vi "Drive_Loop_Control_Loop.vi"(10 "Init Period":i64, 11 "Drive DevRef In":T2={"Sensor Data"={"Gyro Data"={"Gyro RT FIFO"=refnum, "Gyro Current"=0.0, "Gyro Hold"=0.0}, "Encoder Data"={"Encoder RT FIFO"=refnum, "Encoder Current"=0.0, "Encoder Hold"=0.0}, "Camera Data"={"Camera RT FIFO"=refnum, "Camera Current"={" Angle"=0.0, "Valid"=FALSE}}}, "PID Update"=refnum, "RobotDriveDevRef"={"DevStatus"={"status"=FALSE, "code"=0, "source"=""}, "Motors[]"=[], "Square Inputs"=FALSE, "Max Output"=1.0}, "Drive Train"=enum."Tank Drive 2 Motor", "Valid Commands"=[], "Drive Comand Notifier"=refnum, "Command Finished?"=refnum, "Command Canceled"=refnum}) -> ()   [LabVIEW 2016]
doc: "Help file written by FRC Team 836 - The RoboBees\n\nThis VI combines movment commands with various sensor inputs to control the robot as desired.\n\nThis VI uses VIs & Controls from Worcestor Polytechnic Institure (WPI) located in folder:\nC:\\Program Files (x86)\\National Instruments\\LabVIEW 2015\\vi.lib\\Rock Robotics\\WPI\\RobotDrive\n\nThe RobotDrive VI from WPI does the actual moving of the robot. The RobotDriveDevRef control\nwill pass commands to the WPI VI \"WPI_RobotDriveMotors\" via the WPI VI \"WPI_RobotDriveTankDrive\" to acutate the motors.\n\nThe RT FIFOs must be initialized using the \"Drive_Loop_Initialize_w_Help\" VI."
uses:
  <userlib>/836-libraries/Drive/Drive_Code_V2/Drive_Code_Support/Drive_Code_Bundle.ctl
  <userlib>/836-libraries/Drive/Drive_Code_V2/Drive_Code_Support/SensorTypedefs/Sensor_Cluster.ctl
  <userlib>/836-libraries/Drive/Drive_Code_V2/Drive_Code_Support/SensorTypedefs/Camera_Cluster.ctl
  <userlib>/836-libraries/Drive/Drive_Code_V2/Drive_Code_Support/PidClusters/Drive_Code_PID_Bundle.ctl
  <vilib>/Rock Robotics/WPI/RobotDrive/WPI_RobotDriveDevRef.ctl
  <vilib>/Rock Robotics/WPI/MotorControl/WPI_MotorControlDeviceRef.ctl
  <vilib>/Rock Robotics/WPI/MotorControl/WPI_MotorControlType.ctl
  <vilib>/Rock Robotics/SystemInterfaces/DIO/FPGA_DIOPWMChannel.ctl
  <vilib>/Rock Robotics/WPI/PWM/WPI_PWMDeadband.ctl
  <userlib>/836-libraries/Drive/Drive_Code_V2/Drive_Code_Support/DriveTrains/Drive_Trains.ctl
  <userlib>/836-libraries/Drive/Drive_Code_V2/Drive_Code_Support/Command_Sends/Drive_Code_Command_Type.ctl
  <userlib>/836-libraries/Drive/Drive_Code_V2/Drive_Code_Support/Command_Sends/Drive_Code_Command_List.ctl
  <vilib>/Platform/TimedLoop/XDataNode/timing_clust.ctl
  <vilib>/Platform/TimedLoop/XDataNode/nitl_modes.ctl
  <vilib>/Platform/TimedLoop/XDataNode/wakeup.ctl
  <userlib>/836-libraries/Drive/Drive_Code_V2/Drive_Code_Support/DriveTrains/Drive_Values.ctl
  <userlib>/836-libraries/Drive/Drive_Code_V2/Drive_Code_Support/Command_Sends/CommandTypeInfo/DriveContinuousParam.ctl
  <userlib>/836-libraries/Drive/Drive_Code_V2/Drive_Code_Support/Command_Sends/CommandTypeInfo/AngleInfo.ctl
  <userlib>/836-libraries/Drive/Drive_Code_V2/Drive_Code_Support/Command_Sends/CommandTypeInfo/TurnParam.ctl
  <userlib>/836-libraries/Drive/Drive_Code_V2/Drive_Code_Support/Command_Sends/CommandTypeInfo/DriveDistanceParam.ctl
  <userlib>/836-libraries/Drive/Drive_Code_V2/Drive_Code_Support/Command_Sends/CommandTypeInfo/DistanceInfo.ctl
  <userlib>/836-libraries/Drive/Drive_Code_V2/Drive_Code_Support/Command_Sends/CommandTypeInfo/ApproachCameraParam.ctl
  <userlib>/836-libraries/Drive/Drive_Code_V2/Drive_Code_Support/Command_Sends/CommandTypeInfo/UpdatePeriodParam.ctl
  <vilib>/addons/control/pid/pid.llb/PID (DBL).vi
  <vilib>/platform/TimedLoop/XDataNode/XDataNode.xnode
  <vilib>/Platform/TimedLoop/XDataNode/XDNodeRunTimeDep.lvlib
  <vilib>/addons/control/pid/NI_PID_pid.lvlib
panel:
  in  "Init PID Gains":T1={"Yaw, Driving Straight"={"proportional gain (Kc)"=1.0, "integral time (Ti, min)"=0.01, "derivative time (Td, min)"=0.0}, "Yaw, Holding Still"={"proportional gain (Kc)"=1.0, "integral time (Ti, min)"=0.01, "derivative time (Td, min)"=0.0}, "Distance, Driving Straight"={"proportional gain (Kc)"=1.0, "integral time (Ti, min)"=0.01, "derivative time (Td, min)"=0.0}, "Distance, Holding Still"={"proportional gain (Kc)"=1.0, "integral time (Ti, min)"=0.01, "derivative time (Td, min)"=0.0}}
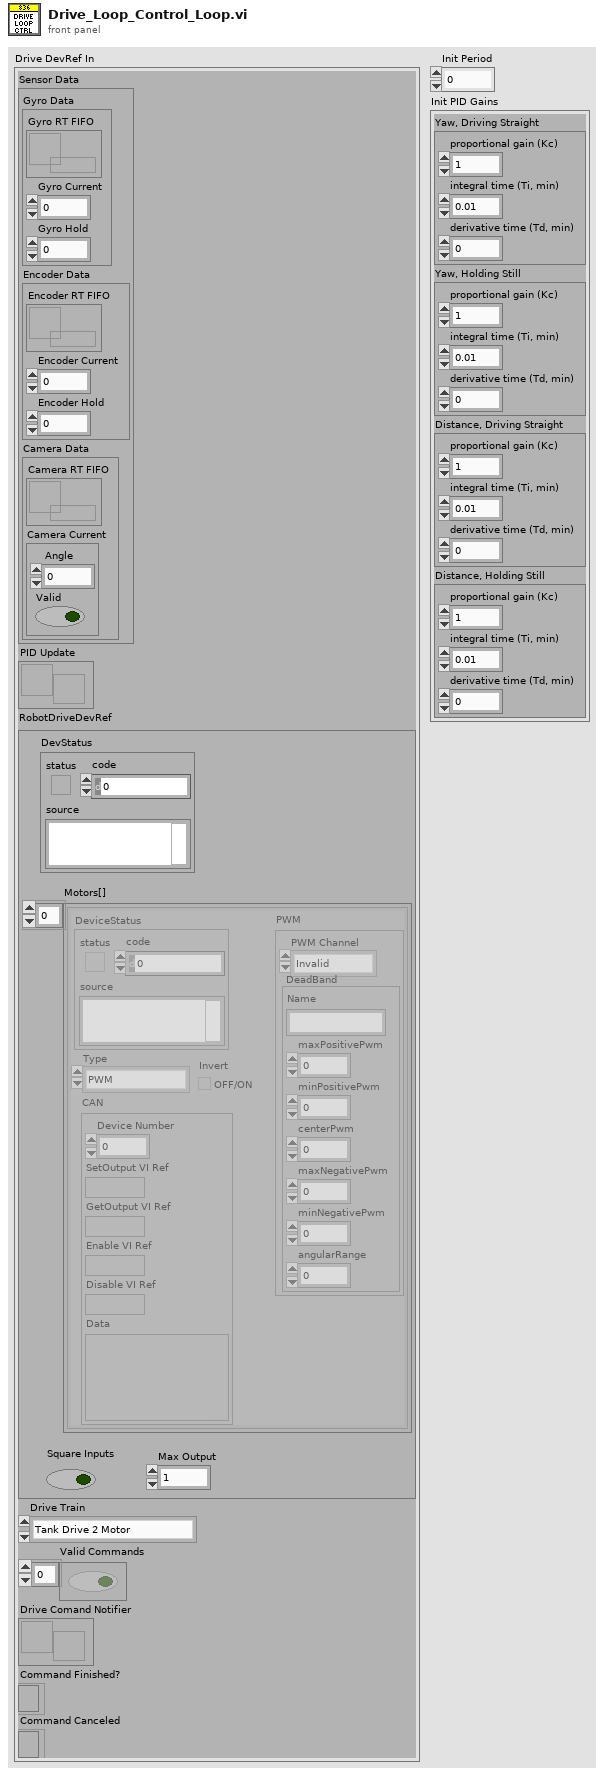
[diagram p1: front panel]
types:
  T1 = typedef "Drive_Code_PID_Bundle.ctl" = cluster{"Yaw, Driving Straight":cluster{"proportional gain (Kc)":dbl, "integral time (Ti, min)":dbl, "derivative time (Td, min)":dbl}, "Yaw, Holding Still":cluster{"proportional gain (Kc)":dbl, "integral time (Ti, min)":dbl, "derivative time (Td, min)":dbl}, "Distance, Driving Straight":cluster{"proportional gain (Kc)":dbl, "integral time (Ti, min)":dbl, "derivative time (Td, min)":dbl}, "Distance, Holding Still":cluster{"proportional gain (Kc)":dbl, "integral time (Ti, min)":dbl, "derivative time (Td, min)":dbl}}
  T2 = typedef "Drive_Code_Bundle.ctl" = cluster{"Sensor Data":T3, "PID Update":refnum<notifier>, "RobotDriveDevRef":T5, "Drive Train":T10, "Valid Commands":bool[], "Drive Comand Notifier":refnum<notifier>, "Command Finished?":refnum<k4>, "Command Canceled":refnum<k4>}
  T3 = typedef "Sensor_Cluster.ctl" = cluster{"Gyro Data":cluster{"Gyro RT FIFO":refnum<k33>, "Gyro Current":dbl, "Gyro Hold":dbl}, "Encoder Data":cluster{"Encoder RT FIFO":refnum<k33>, "Encoder Current":dbl, "Encoder Hold":dbl}, "Camera Data":cluster{"Camera RT FIFO":refnum<k33>, "Camera Current":T4}}
  T4 = typedef "Camera_Cluster.ctl" = cluster{" Angle":dbl, "Valid":bool}
  T5 = typedef "WPI_RobotDriveDevRef.ctl" = cluster{"DevStatus":errorcluster, "Motors[]":T6[], "Square Inputs":bool, "Max Output":dbl}
  T6 = typedef "WPI_MotorControlDeviceRef.ctl" = cluster{"DeviceStatus":errorcluster, "Type":T7, "PWM":cluster{"PWM Channel":T8, "DeadBand":T9}, "CAN":cluster{"Device Number":u8, "SetOutput VI Ref":variant, "GetOutput VI Ref":variant, "Enable VI Ref":variant, "Disable VI Ref":variant, "Data":variant}, "Invert":bool}
  T7 = typedef "WPI_MotorControlType.ctl" = enum16{"PWM", "CAN"}
  T8 = typedef "FPGA_DIOPWMChannel.ctl" = enum8{"PWM 0", "PWM 1", "PWM 2", "PWM 3", "PWM 4", "PWM 5", "PWM 6", "PWM 7", "PWM 8", "PWM 9", "PWM MXP 0", "PWM MXP 1", "PWM MXP 2", "PWM MXP 3", "PWM MXP 4", "PWM MXP 5", "PWM MXP 6", "PWM MXP 7", "PWM MXP 8", "PWM MXP 9", "Invalid"}
  T9 = typedef "WPI_PWMDeadband.ctl" = cluster{"Name":string, "maxPositivePwm":i32, "minPositivePwm":i32, "centerPwm":i32, "maxNegativePwm":i32, "minNegativePwm":i32, "angularRange":u16}
  T10 = typedef "Drive_Trains.ctl" = enum16{"Tank Drive 2 Motor", "Tank Drive 4 Motor", "Mecanum Drive", "Kiwi Drive"}
  T11 = typedef "Drive_Code_Command_List.ctl" = enum16{"Do Nothing", "Tank Drive", "Drive Continuous", "Turn", "Drive Distance", "Hold Position", "Hold Yaw", "Follow Camera", "Turn to Camera", "Approach Camera", "PID Update", "Cheesy Drive", "Update Period"}
  T12 = typedef "Drive_Code_Command_Type.ctl" = cluster{"Command":T11, "Command Params":variant}
  T13 = typedef "XDNodeRunTimeDep.lvlib/timing_clust.ctl" = cluster{"Expected End [f-1]":u64, "Actual End [f-1]":u64, "Finished Late? [f-1]":bool, "Expected End [i-1]":u64, "Actual End [i-1]":u64, "Finished Late? [i-1]":bool, "Expected Start [i]":u64, "Actual Start [i]":u64, "Expected Start [f]":u64, "Actual Start [f]":u64, "Source Name":string, "Structure Name":string, "Period":i64, "Deadline":i64, "Offset":i64, "Start":i64, "Priority":i32, "Timeout":i32, "Mode":T14, "Wakeup Reason":T15, "Error":errorcluster, "Source Type":string, "Secondary Source Type":string, "Global End Time":u64, "Global Start Time":u64, "Frame Duration":u64, "Iteration Duration":u64, "Assigned CPU":i32, "I/O Scan Engine Mode":u32}
  T14 = typedef "XDNodeRunTimeDep.lvlib/nitl_modes.ctl" = enum32{"No Change", "Process missed periods, maintain original phase", "Discard missed periods, maintain original phase", "Process missed periods, ignore original phase", "Discard missed periods, ignore original phase"}
  T15 = typedef "XDNodeRunTimeDep.lvlib/wakeup.ctl" = enum32{"Normal", "Aborted", "Asynchronous wakeup", "Timing source error", "Timed loop error", "Timeout"}
  T16 = typedef "Drive_Values.ctl" = cluster{"Right":dbl, "Left":dbl, "Throttle":dbl, "Wheel":dbl, "Rotation":dbl, "X":dbl, "Y":dbl}
  T17 = typedef "DriveContinuousParam.ctl" = cluster{"Max Turn Power":dbl, "Angle To Drive At":T18, "Foward Power":dbl}
  T18 = typedef "AngleInfo.ctl" = cluster{"Angle":dbl, "Angle Absolute?":bool}
  T19 = typedef "TurnParam.ctl" = cluster{"Max Power":dbl, "Angle To Turn To":T18}
  T20 = typedef "DriveDistanceParam.ctl" = cluster{"Max Turn Power":dbl, "Distance To Drive":T21, "Angle To Drive At":T18, "Max Forward Power":dbl}
  T21 = typedef "DistanceInfo.ctl" = cluster{"Distance":dbl, "Distance Absolute?":bool}
  T22 = typedef "ApproachCameraParam.ctl" = cluster{"Max Turn Power":dbl, "Distance To Drive":T21, "Max Forward Power":dbl}
  T23 = typedef "UpdatePeriodParam.ctl" = cluster{"Period":i64}
  T24 = cluster{"Gyro RT FIFO":refnum<k33>, "Gyro Current":dbl, "Gyro Hold":dbl}
  T25 = cluster{"Encoder RT FIFO":refnum<k33>, "Encoder Current":dbl, "Encoder Hold":dbl}
  T26 = cluster{"Camera RT FIFO":refnum<k33>, "Camera Current":T4}
  T27 = typedef "DrivePidInputs.ctl" = cluster{"EncoderPID":T28, "YawPID":T28}
  T28 = typedef "PidInputs.ctl" = cluster{"Setpoint":dbl, "Process":dbl}
  T29 = typedef "DrivePidRange.ctl" = cluster{"Encoder PID Range":T30, "Yaw PID Range":T30}
  T30 = typedef "PidRange.ctl" = cluster{"Max":dbl, "Min":dbl}
  T31 = cluster{"proportional gain (Kc)":dbl, "integral time (Ti, min)":dbl, "derivative time (Td, min)":dbl}
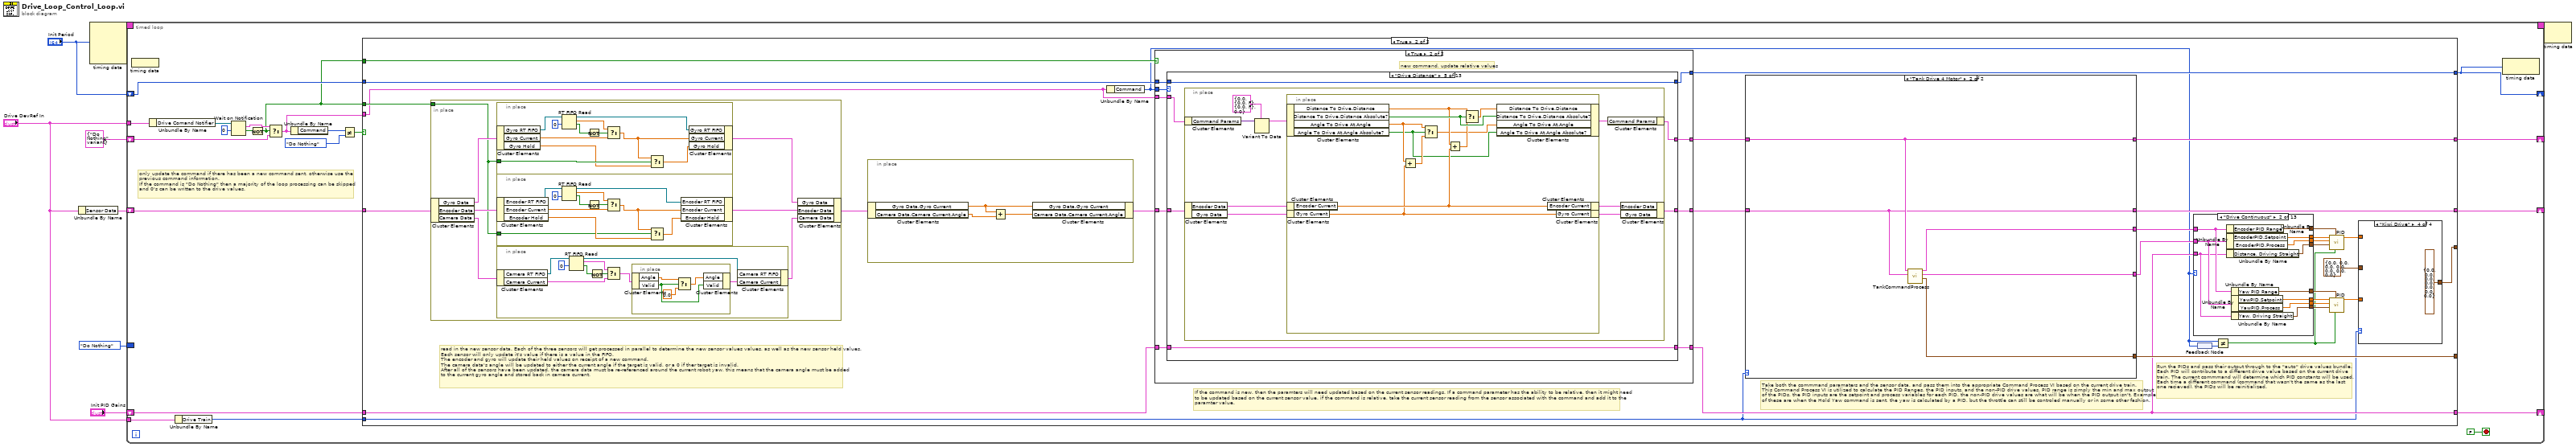
[diagram p0: block diagram]
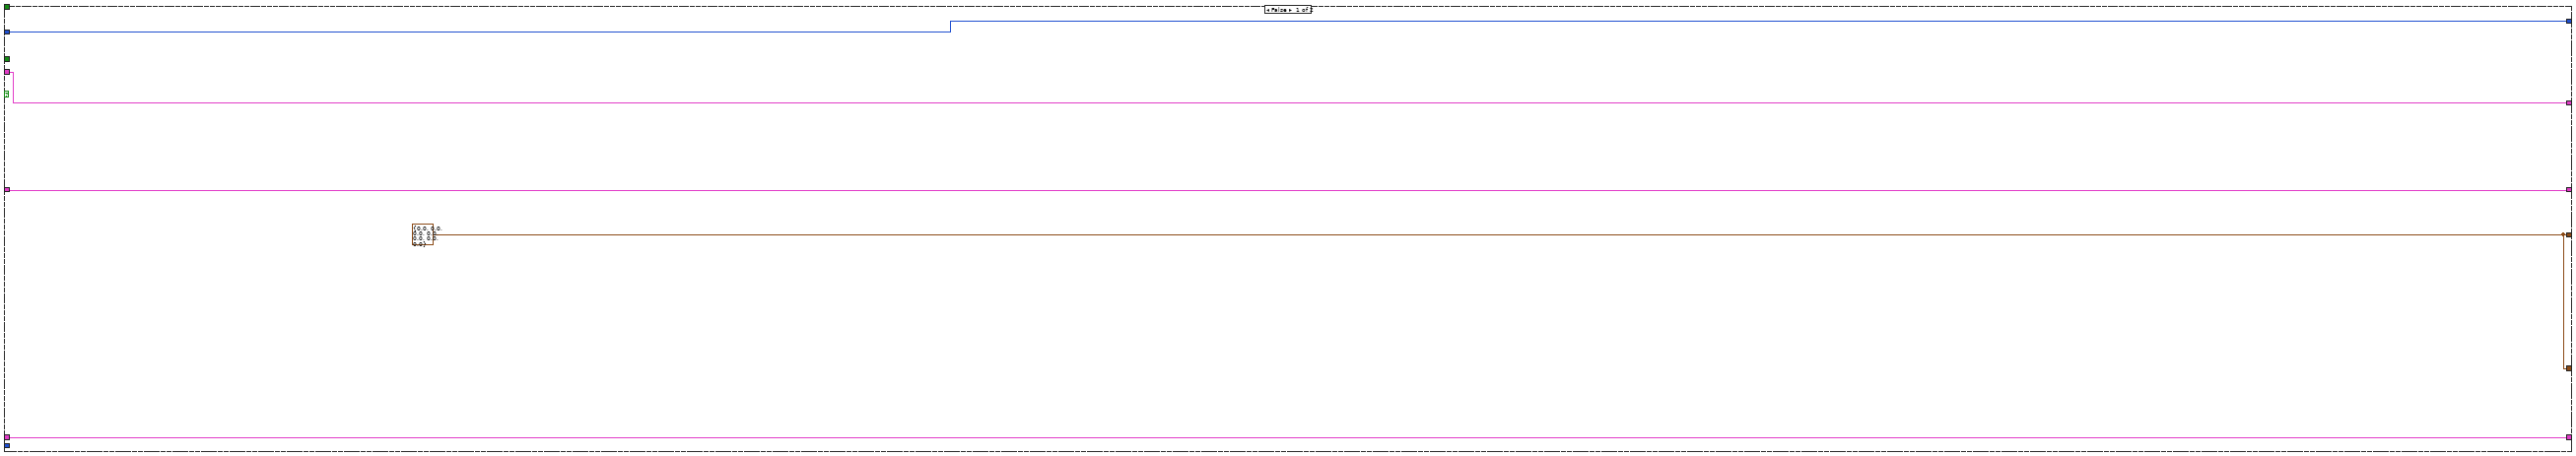
[diagram p2: hidden frame]
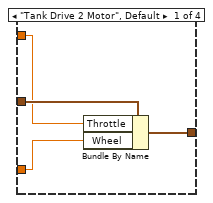
[diagram p3: hidden frame]
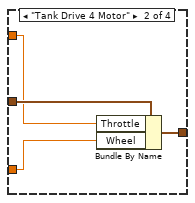
[diagram p4: hidden frame]
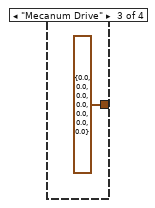
[diagram p5: hidden frame]
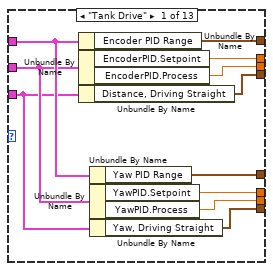
[diagram p6: hidden frame]
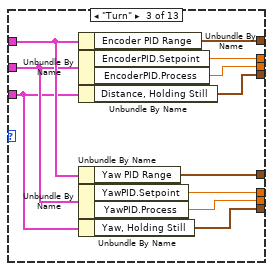
[diagram p7: hidden frame]
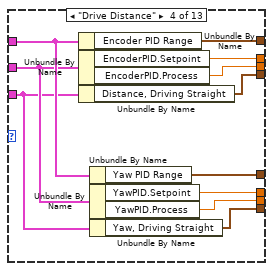
[diagram p8: hidden frame]
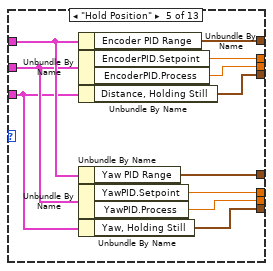
[diagram p9: hidden frame]
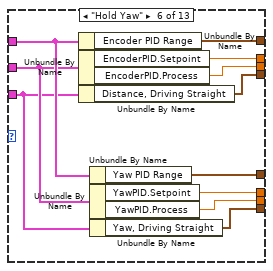
[diagram p10: hidden frame]
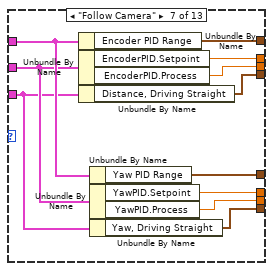
[diagram p11: hidden frame]
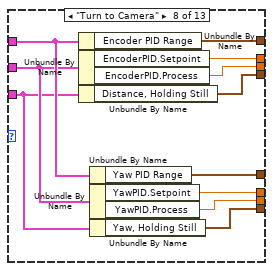
[diagram p12: hidden frame]
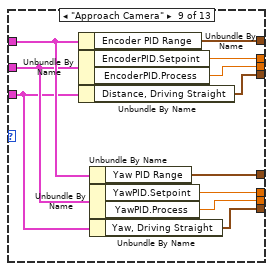
[diagram p13: hidden frame]
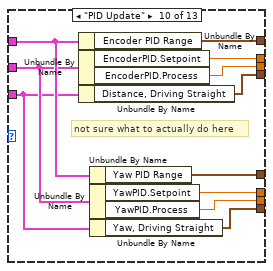
[diagram p14: hidden frame]
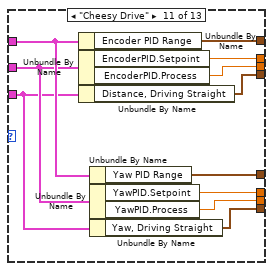
[diagram p15: hidden frame]
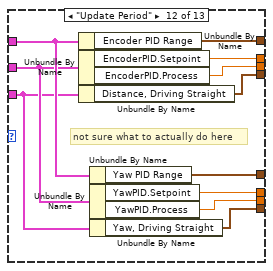
[diagram p16: hidden frame]
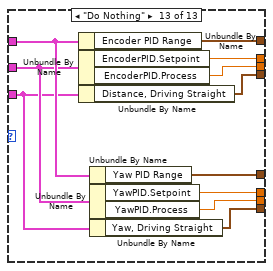
[diagram p17: hidden frame]
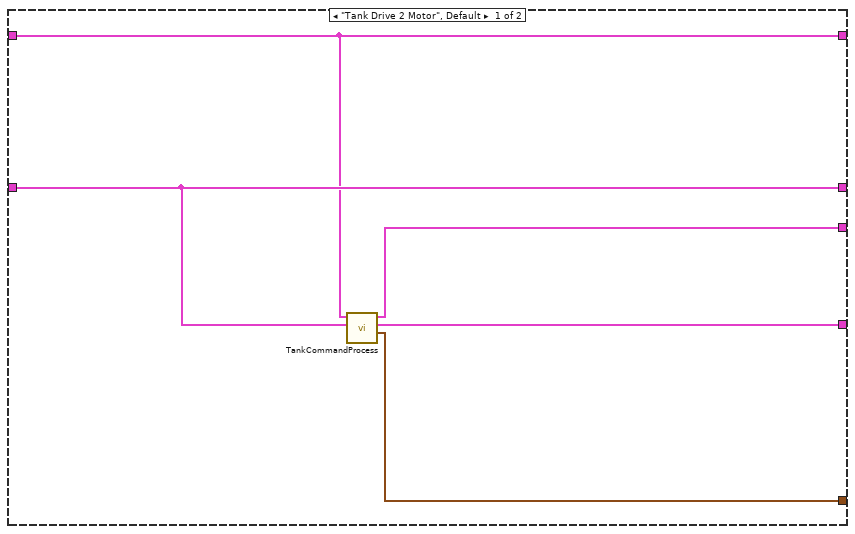
[diagram p18: hidden frame]
diagram:
  n1 = Unbundle By Name("Drive DevRef In") -> ("Sensor Data"=w3:T3)
  n2 = node-c288("Init Period") -> (w8:T13)  [unwired: 3 in]
  n3 = timed-loop {
    timing: w8 -> [_]
    timing-out: [_] -> w7
    shift-right: [w17] -> _
    shift-left: "Init Period" -> [w18]
    tunnel: "Drive DevRef In" -> [w20]
    shift-right: [w16] -> _
    shift-left: T12 {"Command"=enum."Do Nothing", "Command Params"=variant} ("Command Type") -> [w24]
    shift-right: [w13] -> _
    shift-left: "Init PID Gains" -> [w14]
    shift-right: [w15] -> _
    shift-left: w3 -> [w19]
    tunnel: "Drive DevRef In" -> [w10]
    border: Drive_Code_Command_List."Do Nothing" ("Command") -> [_]
    stop <- FALSE stop-if-true
    # "only update the command if there has been a new command sent, otherwise use the\nprevious command information.\nIf the command is \"Do Nothing\" then a majority of the loop processing can be skipped\nand 0's can be written to the drive values."
    n4 = node-c288() -> ()  [unwired: 1 in]
    n5 = Unbundle By Name(w20) -> ("Drive Comand Notifier"=w28:refnum<notifier>)
    n6 = Unbundle By Name(w10) -> ("Drive Train"=w9:T10)
    n7 = Wait on Notification(notifier=w28, timeout in ms (-1)=0) -> (notification=w25:T12, timed out?=w26:bool)  [unwired: 2 in, 2 out]
    n8 = Not(x=w26) -> (.not. x?=w11:bool)
    n9 = Select(t=w25, s=w11, f=w24) -> (s? t:f=w21:T12)
    n10 = Unbundle By Name(w21) -> ("Command"=w12:T11)
    n11 = Not Equal?(x=w12, y=Drive_Code_Command_List."Do Nothing") -> (x != y?=w22:bool)
    n12 = case shown="True" w22 {
      tunnel: [w30 w35] -> _
      tunnel: w21 -> [w33 w64]
      tunnel: w11 -> [_ w67]
      tunnel: w19 -> [w32 w66]
      tunnel: w18 -> [w34 w65]
      tunnel: [w34 w63] -> w17
      tunnel: [w33 w57] -> w16
      tunnel: [w32 w56] -> w15
      tunnel: w14 -> [w31 w62]
      tunnel: [w31 w48] -> w13
      tunnel: w11 -> [_ w43]
      tunnel: w9 -> [_ w38]
      tunnel: [w30 w55] -> _
      frame False {
        w30 = T16 {"Right"=0.0, "Left"=0.0, "Throttle"=0.0, "Wheel"=0.0, "Rotation"=0.0, "X"=0.0, "Y"=0.0}
      }
      frame True {
        # "Run the PIDs and pass their output through to the \"auto\" drive values bundle.\nEach PID will contribute to a different drive value based on the current drive\ntrain. The current commmand will determine which PID constants will be used.\nEach time a different command (command that wasn't the same as the last \none recieved), the PIDs will be reinitialized."
        # "Take both the commmand paramaters and the sensor data, and pass them into the appropriate Command Process VI based on the current drive train.\nThis Command Process VI is utilized to calculate the PID Ranges, the PID inputs, and the non-PID drive values. PID range is simply the min and max output\nof the PIDs, the PID inputs are the setpoint and process variables for each PID, the non-PID drive values are what will be when the PID output isn't. Examples\nof these are when the Hold Yaw command is sent, the yaw is calculated by a PID, but the throttle can still be controled manually or in some other fashion."
        # "If the command is new, then the paramters will need updated based on the current sensor readings. If a command parameter has the ability to be relative, then it might need\nto be updated based on the current sensor value. if the command is relative, take the current sensor reading from the sensor associated with the command and add it to the\nparamter value."
        # "read in the new sensor data. Each of the three sensors will get processed in parallel to determine the new sensor values values, as well as the new sensor held values.\nEach sensor will only update it's value if there is a value in the FIFO.\nThe encoder and gyro will update their held values on receipt of a new command.\nThe camera data's angle will be updated to either the current angle if the target is valid, or a 0 if ther target is invalid.\nAfter all of the sensors have been updated, the camera data must be re-referenced around the current robot yaw, this means that the camera angle must be added\nto the current gyro angle and stored back in camera current."
        n13 = in-place {
          in-place-border: w67 -> [w366]
          n14 = in-place-cluster #1(w66) -> ("Gyro Data"=w372:T24, "Encoder Data"=w370:T25, "Camera Data"=w368:T26)
          n15 = in-place {
            in-place-border: w366 -> [w399]
            n16 = in-place-cluster #2(w372) -> ("Gyro RT FIFO"=w407:refnum<k33>, "Gyro Current"=w401:dbl, "Gyro Hold"=w397:dbl)
            n17 = RT FIFO Read(0:w407, 2:0 ("timeout in ms (0)")) -> (8:w405:refnum<k33>, 9:w403:dbl, 10:w404:bool)  [unwired: 2 in, 2 out]
            n18 = Not(x=w404) -> (.not. x?=w402:bool)
            n19 = Select(t=w403, s=w402, f=w401) -> (s? t:f=w398:dbl)
            n20 = Select(t=w398, s=w399, f=w397) -> (s? t:f=w400:dbl)
            n21 = in-place-cluster #2("Gyro RT FIFO"=w405, "Gyro Current"=w398, "Gyro Hold"=w400) -> (w371:T24)
          }
          n22 = in-place {
            in-place-border: w366 -> [w386]
            n23 = in-place-cluster #3(w370) -> ("Encoder RT FIFO"=w396:refnum<k33>, "Encoder Current"=w390:dbl, "Encoder Hold"=w387:dbl)
            n24 = RT FIFO Read(0:w396, 2:0 ("timeout in ms (0)")) -> (8:w394:refnum<k33>, 9:w392:dbl, 10:w393:bool)  [unwired: 2 in, 2 out]
            n25 = Not(x=w393) -> (.not. x?=w391:bool)
            n26 = Select(t=w392, s=w391, f=w390) -> (s? t:f=w388:dbl)
            n27 = Select(t=w388, s=w386, f=w387) -> (s? t:f=w389:dbl)
            n28 = in-place-cluster #3("Encoder RT FIFO"=w394, "Encoder Current"=w388, "Encoder Hold"=w389) -> (w369:T25)
          }
          n29 = in-place {
            n30 = in-place-cluster #4(w368) -> ("Camera RT FIFO"=w381:refnum<k33>, "Camera Current"=w375:T4)
            n31 = RT FIFO Read(0:w381, 2:0 ("timeout in ms (0)")) -> (8:w379:refnum<k33>, 9:w376:T4, 10:w378:bool)  [unwired: 2 in, 2 out]
            n32 = Not(x=w378) -> (.not. x?=w377:bool)
            n33 = Select(t=w376, s=w377, f=w375) -> (s? t:f=w374:T4)
            n34 = in-place {
              n35 = in-place-cluster #5(w374) -> ("Angle"=w385:dbl, "Valid"=w383:bool)
              n36 = Select(t=w385, s=w383, f=0.0) -> (s? t:f=w384:dbl)
              n37 = in-place-cluster #5("Angle"=w384, "Valid"=w383) -> (w373:T4)
            }
            n38 = in-place-cluster #4("Camera RT FIFO"=w379, "Camera Current"=w373) -> (w367:T26)
          }
          n39 = in-place-cluster #1("Gyro Data"=w371, "Encoder Data"=w369, "Camera Data"=w367) -> (w59:T3)
        }
        n40 = in-place {
          n41 = in-place-cluster #6(w59) -> ("Gyro Data.Gyro Current"=w223:dbl, "Camera Data.Camera Current.Angle"=w221:dbl)
          n42 = Add(x=w223, y=w221) -> (x+y=w222:dbl)
          n43 = in-place-cluster #6("Gyro Data.Gyro Current"=w223, "Camera Data.Camera Current.Angle"=w222) -> (w58:T3)
        }
        n44 = Unbundle By Name(w64) -> ("Command"=w41:T11)
        n45 = case shown="True" w43 {
          tunnel: w65 -> [w234 w246]
          tunnel: w58 -> [w236 w245]
          tunnel: w41 -> [_ w244]
          tunnel: w64 -> [w237 w243]
          tunnel: [w234 w242] -> w63
          tunnel: [w236 w241] -> w60
          tunnel: [w237 w240] -> w61
          tunnel: [w235 w239] -> w48
          tunnel: w62 -> [w235 w238]
          frame False {
          }
          frame True {
            # "new command, update relative values"
            n46 = case shown="\"Drive Distance\"" w244 {
              tunnel: w246 -> [w250 w254 w260 w277 w294 w316 w320 w324 w328 w334 w352 _ w361]
              tunnel: w245 -> [w248 w251 w258 w274 w291 w313 w317 w321 w325 w331 w349 w355 w364]
              tunnel: w243 -> [w247 w252 w259 w275 w292 w314 w318 w322 w326 w332 w350 w354 w363]
              tunnel: [w250 w254 w260 w277 w294 w316 w320 w324 w328 w334 w352 w356 w361] -> w242
              tunnel: [w248 w251 w256 w272 w289 w313 w317 w321 w325 w330 w349 w355 w364] -> w241
              tunnel: [w247 w252 w257 w273 w290 w314 w318 w322 w326 w329 w350 w354 w363] -> w240
              tunnel: [w249 w253 w255 w276 w293 w315 w319 w323 w327 w333 w351 w353 w360] -> w239
              tunnel: w238 -> [w249 w253 w255 w276 w293 w315 w319 w323 w327 w333 w351 w353 _]
              frame "Do Nothing", Default {
              }
              frame "Tank Drive" {
                # "no portion of this command's params need to be updated because they can't be relative to anything."
              }
              frame "Drive Continuous" {
                n47 = in-place {
                  n48 = in-place-cluster #7(w259) -> ("Command Params"=w266:variant)
                  n49 = in-place-cluster #8(w258) -> ("Gyro Data"=w262:T24)
                  n50 = Variant To Data(type=T17 {"Max Turn Power"=0.0, "Angle To Drive At"={"Angle"=0.0, "Angle Absolute?"=FALSE}, "Foward Power"=0.0} ("Drive Continuous Param"), Variant=w266) -> (data=w264:T17)  [unwired: 1 in, 1 out]
                  n51 = in-place {
                    n52 = in-place-cluster #9(w264) -> ("Angle To Drive At.Angle"=w269:dbl, "Angle To Drive At.Angle Absolute?"=w270:bool)
                    n53 = in-place-cluster #10(w262) -> ("Gyro Current"=w267:dbl)
                    n54 = Add(x=w269, y=w267) -> (x+y=w268:dbl)
                    n55 = Select(t=w269, s=w270, f=w268) -> (s? t:f=w271:dbl)
                    n56 = in-place-cluster #9("Angle To Drive At.Angle"=w271, "Angle To Drive At.Angle Absolute?"=w270) -> (w263:T17)
                    n57 = in-place-cluster #10("Gyro Current"=w267) -> (w261:T24)
                  }
                  n58 = in-place-cluster #7("Command Params"=w263) -> (w257:T12)
                  n59 = in-place-cluster #8("Gyro Data"=w261) -> (w256:T3)
                }
              }
              frame "Turn" {
                n60 = in-place {
                  n61 = in-place-cluster #11(w275) -> ("Command Params"=w283:variant)
                  n62 = in-place-cluster #12(w274) -> ("Gyro Data"=w280:T24)
                  n63 = Variant To Data(type=T19 {"Max Power"=0.0, "Angle To Turn To"={"Angle"=0.0, "Angle Absolute?"=FALSE}} ("Turn Param"), Variant=w283) -> (data=w281:T19)  [unwired: 1 in, 1 out]
                  n64 = in-place {
                    n65 = in-place-cluster #13(w281) -> ("Angle To Turn To.Angle"=w284:dbl, "Angle To Turn To.Angle Absolute?"=w286:bool)
                    n66 = in-place-cluster #14(w280) -> ("Gyro Current"=w285:dbl)
                    n67 = Add(x=w284, y=w285) -> (x+y=w288:dbl)
                    n68 = Select(t=w284, s=w286, f=w288) -> (s? t:f=w287:dbl)
                    n69 = in-place-cluster #13("Angle To Turn To.Angle"=w287, "Angle To Turn To.Angle Absolute?"=w286) -> (w278:T19)
                    n70 = in-place-cluster #14("Gyro Current"=w285) -> (w279:T24)
                  }
                  n71 = in-place-cluster #11("Command Params"=w278) -> (w273:T12)
                  n72 = in-place-cluster #12("Gyro Data"=w279) -> (w272:T3)
                }
              }
              frame "Drive Distance" {
                n73 = in-place {
                  n74 = in-place-cluster #15(w292) -> ("Command Params"=w302:variant)
                  n75 = in-place-cluster #16(w291) -> ("Encoder Data"=w299:T25, "Gyro Data"=w298:T24)
                  n76 = Variant To Data(type=T20 {"Max Turn Power"=0.0, "Distance To Drive"={"Distance"=0.0, "Distance Absolute?"=FALSE}, "Angle To Drive At"={"Angle"=0.0, "Angle Absolute?"=FALSE}, "Max Forward Power"=0.0} ("Drive Distance Param"), Variant=w302) -> (data=w300:T20)  [unwired: 1 in, 1 out]
                  n77 = in-place {
                    n78 = in-place-cluster #17(w300) -> ("Distance To Drive.Distance"=w310:dbl, "Distance To Drive.Distance Absolute?"=w311:bool, "Angle To Drive At.Angle"=w306:dbl, "Angle To Drive At.Angle Absolute?"=w303:bool)
                    n79 = in-place-cluster #18(w299) -> ("Encoder Current"=w309:dbl)
                    n80 = in-place-cluster #19(w298) -> ("Gyro Current"=w305:dbl)
                    n81 = Add(x=w306, y=w305) -> (x+y=w307:dbl)
                    n82 = Select(t=w306, s=w303, f=w307) -> (s? t:f=w304:dbl)
                    n83 = Add(x=w310, y=w309) -> (x+y=w308:dbl)
                    n84 = Select(t=w310, s=w311, f=w308) -> (s? t:f=w312:dbl)
                    n85 = in-place-cluster #17("Distance To Drive.Distance"=w312, "Distance To Drive.Distance Absolute?"=w311, "Angle To Drive At.Angle"=w304, "Angle To Drive At.Angle Absolute?"=w303) -> (w295:T20)
                    n86 = in-place-cluster #18("Encoder Current"=w309) -> (w297:T25)
                    n87 = in-place-cluster #19("Gyro Current"=w305) -> (w296:T24)
                  }
                  n88 = in-place-cluster #15("Command Params"=w295) -> (w290:T12)
                  n89 = in-place-cluster #16("Encoder Data"=w297, "Gyro Data"=w296) -> (w289:T3)
                }
              }
              frame "Hold Position" {
                # "no portion of this command's params need to be updated because they can't be relative to anything."
              }
              frame "Hold Yaw" {
                # "no portion of this command's params need to be updated because they can't be relative to anything."
              }
              frame "Follow Camera" {
                # "no portion of this command's params need to be updated because they can't be relative to anything."
              }
              frame "Turn to Camera" {
                # "no portion of this command's params need to be updated because they can't be relative to anything."
              }
              frame "Approach Camera" {
                n90 = in-place {
                  n91 = in-place-cluster #20(w332) -> ("Command Params"=w342:variant)
                  n92 = in-place-cluster #21(w331) -> ("Encoder Data"=w340:T25, "Gyro Data"=w339:T24)
                  n93 = Variant To Data(type=T22 {"Max Turn Power"=0.0, "Distance To Drive"={"Distance"=0.0, "Distance Absolute?"=FALSE}, "Max Forward Power"=0.0} ("Approach Camera Param"), Variant=w342) -> (data=w341:T22)  [unwired: 1 in, 1 out]
                  n94 = in-place {
                    n95 = in-place-cluster #22(w341) -> ("Distance To Drive.Distance"=w346:dbl, "Distance To Drive.Distance Absolute?"=w347:bool)
                    n96 = in-place-cluster #23(w340) -> ("Encoder Current"=w345:dbl)
                    n97 = in-place-cluster #24(w339) -> ("Gyro Current"=w343:dbl)
                    n98 = Add(x=w346, y=w345) -> (x+y=w344:dbl)
                    n99 = Select(t=w346, s=w347, f=w344) -> (s? t:f=w348:dbl)
                    n100 = in-place-cluster #22("Distance To Drive.Distance"=w348, "Distance To Drive.Distance Absolute?"=w347) -> (w336:T22)
                    n101 = in-place-cluster #23("Encoder Current"=w345) -> (w338:T25)
                    n102 = in-place-cluster #24("Gyro Current"=w343) -> (w337:T24)
                  }
                  n103 = in-place-cluster #20("Command Params"=w336) -> (w329:T12)
                  n104 = in-place-cluster #21("Encoder Data"=w338, "Gyro Data"=w337) -> (w330:T3)
                }
              }
              frame "Cheesy Drive" {
                # "no portion of this command's params need to be updated because they can't be relative to anything."
              }
              frame "Update Period" {
                # "no portion of this command's params need to be updated because they can't be relative to anything."
                n105 = Unbundle By Name(w354) -> ("Command Params"=w359:variant)
                n106 = Variant To Data(type=T23 {"Period"=0} ("Update Period Param"), Variant=w359) -> (data=w357:T23)  [unwired: 1 in, 1 out]
                n107 = Unbundle By Name(w357) -> ("Period"=w356:i64)
              }
              frame "PID Update" {
                # "no portion of this command's params need to be updated because they can't be relative to anything."
                n108 = Unbundle By Name(w363) -> ("Command Params"=w365:variant)
                n109 = Variant To Data(type=T1 {"Yaw, Driving Straight"={"proportional gain (Kc)"=1.0, "integral time (Ti, min)"=0.01, "derivative time (Td, min)"=0.0}, "Yaw, Holding Still"={"proportional gain (Kc)"=1.0, "integral time (Ti, min)"=0.01, "derivative time (Td, min)"=0.0}, "Distance, Driving Straight"={"proportional gain (Kc)"=1.0, "integral time (Ti, min)"=0.01, "derivative time (Td, min)"=0.0}, "Distance, Holding Still"={"proportional gain (Kc)"=1.0, "integral time (Ti, min)"=0.01, "derivative time (Td, min)"=0.0}} ("PID Gains"), Variant=w365) -> (data=w360:T1)  [unwired: 1 in, 1 out]
              }
            }
          }
        }
        n110 = case shown="\"Tank Drive 4 Motor\"" w38 {
          tunnel: w61 -> [w224 w230]
          tunnel: w60 -> [w225 w229]
          tunnel: [w228 w233] -> w50
          tunnel: [w227 w232] -> w49
          tunnel: [w226 w231] -> w55
          tunnel: [w224 w230] -> w57
          tunnel: [w225 w229] -> w56
          frame "Tank Drive 2 Motor", Default {
            n111 = call <userlib>:"TankCommandProcess.vi"("Sensor Cluster"=w225, "Command"=w224) -> ("Non PID Drive Values"=w226:T16, "PID Values"=w227:T27, "PID Ranges"=w228:T29)  [unwired: 7 in]
          }
          frame "Tank Drive 4 Motor" {
            n112 = call <userlib>:"TankCommandProcess.vi"("Sensor Cluster"=w229, "Command"=w230) -> ("Non PID Drive Values"=w231:T16, "PID Values"=w232:T27, "PID Ranges"=w233:T29)  [unwired: 7 in]
          }
        }
        n113 = case shown="\"Drive Continuous\"" w41 {
          tunnel: [w88 w99 w110 w121 w132 w143 w154 w165 w176 w187 w198 w209 w220] -> w54
          tunnel: [w87 w98 w109 w120 w131 w142 w153 w164 w175 w186 w197 w208 w219] -> w53
          tunnel: [w86 w97 w108 w119 w130 w141 w152 w163 w174 w185 w196 w207 w218] -> w52
          tunnel: [w85 w96 w107 w118 w129 w140 w151 w162 w173 w184 w195 w206 w217] -> w51
          tunnel: w50 -> [w84 w95 w106 w117 w128 w139 w150 w161 w172 w183 w194 w205 w216]
          tunnel: w49 -> [w83 w94 w105 w116 w127 w138 w149 w160 w171 w182 w193 w204 w215]
          tunnel: w48 -> [w82 w93 w104 w115 w126 w137 w148 w159 w170 w181 w192 w203 w214]
          tunnel: [w81 w92 w103 w114 w125 w136 w147 w158 w169 w180 w191 w202 w213] -> w47
          tunnel: [w80 w91 w102 w113 w124 w135 w146 w157 w168 w179 w190 w201 w212] -> w46
          tunnel: [w79 w90 w101 w112 w123 w134 w145 w156 w167 w178 w189 w200 w211] -> w45
          tunnel: [w78 w89 w100 w111 w122 w133 w144 w155 w166 w177 w188 w199 w210] -> w44
          frame "Tank Drive" {
            n114 = Unbundle By Name(w84) -> ("Encoder PID Range"=w88:T30)
            n115 = Unbundle By Name(w83) -> ("EncoderPID.Setpoint"=w87:dbl, "EncoderPID.Process"=w86:dbl)
            n116 = Unbundle By Name(w82) -> ("Distance, Driving Straight"=w85:T31)
            n117 = Unbundle By Name(w84) -> ("Yaw PID Range"=w78:T30)
            n118 = Unbundle By Name(w83) -> ("YawPID.Setpoint"=w81:dbl, "YawPID.Process"=w80:dbl)
            n119 = Unbundle By Name(w82) -> ("Yaw, Driving Straight"=w79:T31)
          }
          frame "Drive Continuous" {
            n120 = Unbundle By Name(w95) -> ("Encoder PID Range"=w99:T30)
            n121 = Unbundle By Name(w94) -> ("EncoderPID.Setpoint"=w98:dbl, "EncoderPID.Process"=w97:dbl)
            n122 = Unbundle By Name(w93) -> ("Distance, Driving Straight"=w96:T31)
            n123 = Unbundle By Name(w95) -> ("Yaw PID Range"=w89:T30)
            n124 = Unbundle By Name(w94) -> ("YawPID.Setpoint"=w92:dbl, "YawPID.Process"=w91:dbl)
            n125 = Unbundle By Name(w93) -> ("Yaw, Driving Straight"=w90:T31)
          }
          frame "Turn" {
            n126 = Unbundle By Name(w106) -> ("Encoder PID Range"=w110:T30)
            n127 = Unbundle By Name(w105) -> ("EncoderPID.Setpoint"=w109:dbl, "EncoderPID.Process"=w108:dbl)
            n128 = Unbundle By Name(w104) -> ("Distance, Holding Still"=w107:T31)
            n129 = Unbundle By Name(w106) -> ("Yaw PID Range"=w100:T30)
            n130 = Unbundle By Name(w105) -> ("YawPID.Setpoint"=w103:dbl, "YawPID.Process"=w102:dbl)
            n131 = Unbundle By Name(w104) -> ("Yaw, Holding Still"=w101:T31)
          }
          frame "Drive Distance" {
            n132 = Unbundle By Name(w117) -> ("Encoder PID Range"=w121:T30)
            n133 = Unbundle By Name(w116) -> ("EncoderPID.Setpoint"=w120:dbl, "EncoderPID.Process"=w119:dbl)
            n134 = Unbundle By Name(w115) -> ("Distance, Driving Straight"=w118:T31)
            n135 = Unbundle By Name(w117) -> ("Yaw PID Range"=w111:T30)
            n136 = Unbundle By Name(w116) -> ("YawPID.Setpoint"=w114:dbl, "YawPID.Process"=w113:dbl)
            n137 = Unbundle By Name(w115) -> ("Yaw, Driving Straight"=w112:T31)
          }
          frame "Hold Position" {
            n138 = Unbundle By Name(w128) -> ("Encoder PID Range"=w132:T30)
            n139 = Unbundle By Name(w127) -> ("EncoderPID.Setpoint"=w131:dbl, "EncoderPID.Process"=w130:dbl)
            n140 = Unbundle By Name(w126) -> ("Distance, Holding Still"=w129:T31)
            n141 = Unbundle By Name(w128) -> ("Yaw PID Range"=w122:T30)
            n142 = Unbundle By Name(w127) -> ("YawPID.Setpoint"=w125:dbl, "YawPID.Process"=w124:dbl)
            n143 = Unbundle By Name(w126) -> ("Yaw, Holding Still"=w123:T31)
          }
          frame "Hold Yaw" {
            n144 = Unbundle By Name(w139) -> ("Encoder PID Range"=w143:T30)
            n145 = Unbundle By Name(w138) -> ("EncoderPID.Setpoint"=w142:dbl, "EncoderPID.Process"=w141:dbl)
            n146 = Unbundle By Name(w137) -> ("Distance, Driving Straight"=w140:T31)
            n147 = Unbundle By Name(w139) -> ("Yaw PID Range"=w133:T30)
            n148 = Unbundle By Name(w138) -> ("YawPID.Setpoint"=w136:dbl, "YawPID.Process"=w135:dbl)
            n149 = Unbundle By Name(w137) -> ("Yaw, Driving Straight"=w134:T31)
          }
          frame "Follow Camera" {
            n150 = Unbundle By Name(w150) -> ("Encoder PID Range"=w154:T30)
            n151 = Unbundle By Name(w149) -> ("EncoderPID.Setpoint"=w153:dbl, "EncoderPID.Process"=w152:dbl)
            n152 = Unbundle By Name(w148) -> ("Distance, Driving Straight"=w151:T31)
            n153 = Unbundle By Name(w150) -> ("Yaw PID Range"=w144:T30)
            n154 = Unbundle By Name(w149) -> ("YawPID.Setpoint"=w147:dbl, "YawPID.Process"=w146:dbl)
            n155 = Unbundle By Name(w148) -> ("Yaw, Driving Straight"=w145:T31)
          }
          frame "Turn to Camera" {
            n156 = Unbundle By Name(w161) -> ("Encoder PID Range"=w165:T30)
            n157 = Unbundle By Name(w160) -> ("EncoderPID.Setpoint"=w164:dbl, "EncoderPID.Process"=w163:dbl)
            n158 = Unbundle By Name(w159) -> ("Distance, Holding Still"=w162:T31)
            n159 = Unbundle By Name(w161) -> ("Yaw PID Range"=w155:T30)
            n160 = Unbundle By Name(w160) -> ("YawPID.Setpoint"=w158:dbl, "YawPID.Process"=w157:dbl)
            n161 = Unbundle By Name(w159) -> ("Yaw, Holding Still"=w156:T31)
          }
          frame "Approach Camera" {
            n162 = Unbundle By Name(w172) -> ("Encoder PID Range"=w176:T30)
            n163 = Unbundle By Name(w171) -> ("EncoderPID.Setpoint"=w175:dbl, "EncoderPID.Process"=w174:dbl)
            n164 = Unbundle By Name(w170) -> ("Distance, Driving Straight"=w173:T31)
            n165 = Unbundle By Name(w172) -> ("Yaw PID Range"=w166:T30)
            n166 = Unbundle By Name(w171) -> ("YawPID.Setpoint"=w169:dbl, "YawPID.Process"=w168:dbl)
            n167 = Unbundle By Name(w170) -> ("Yaw, Driving Straight"=w167:T31)
          }
          frame "PID Update" {
            # "not sure what to actually do here"
            n168 = Unbundle By Name(w183) -> ("Encoder PID Range"=w187:T30)
            n169 = Unbundle By Name(w182) -> ("EncoderPID.Setpoint"=w186:dbl, "EncoderPID.Process"=w185:dbl)
            n170 = Unbundle By Name(w181) -> ("Distance, Driving Straight"=w184:T31)
            n171 = Unbundle By Name(w183) -> ("Yaw PID Range"=w177:T30)
            n172 = Unbundle By Name(w182) -> ("YawPID.Setpoint"=w180:dbl, "YawPID.Process"=w179:dbl)
            n173 = Unbundle By Name(w181) -> ("Yaw, Driving Straight"=w178:T31)
          }
          frame "Cheesy Drive" {
            n174 = Unbundle By Name(w194) -> ("Encoder PID Range"=w198:T30)
            n175 = Unbundle By Name(w193) -> ("EncoderPID.Setpoint"=w197:dbl, "EncoderPID.Process"=w196:dbl)
            n176 = Unbundle By Name(w192) -> ("Distance, Driving Straight"=w195:T31)
            n177 = Unbundle By Name(w194) -> ("Yaw PID Range"=w188:T30)
            n178 = Unbundle By Name(w193) -> ("YawPID.Setpoint"=w191:dbl, "YawPID.Process"=w190:dbl)
            n179 = Unbundle By Name(w192) -> ("Yaw, Driving Straight"=w189:T31)
          }
          frame "Update Period" {
            # "not sure what to actually do here"
            n180 = Unbundle By Name(w205) -> ("Encoder PID Range"=w209:T30)
            n181 = Unbundle By Name(w204) -> ("EncoderPID.Setpoint"=w208:dbl, "EncoderPID.Process"=w207:dbl)
            n182 = Unbundle By Name(w203) -> ("Distance, Driving Straight"=w206:T31)
            n183 = Unbundle By Name(w205) -> ("Yaw PID Range"=w199:T30)
            n184 = Unbundle By Name(w204) -> ("YawPID.Setpoint"=w202:dbl, "YawPID.Process"=w201:dbl)
            n185 = Unbundle By Name(w203) -> ("Yaw, Driving Straight"=w200:T31)
          }
          frame "Do Nothing" {
            n186 = Unbundle By Name(w216) -> ("Encoder PID Range"=w220:T30)
            n187 = Unbundle By Name(w215) -> ("EncoderPID.Setpoint"=w219:dbl, "EncoderPID.Process"=w218:dbl)
            n188 = Unbundle By Name(w214) -> ("Distance, Driving Straight"=w217:T31)
            n189 = Unbundle By Name(w216) -> ("Yaw PID Range"=w210:T30)
            n190 = Unbundle By Name(w215) -> ("YawPID.Setpoint"=w213:dbl, "YawPID.Process"=w212:dbl)
            n191 = Unbundle By Name(w214) -> ("Yaw, Driving Straight"=w211:T31)
          }
        }
        n192 = feedback-in #25(w41) -> ()
        n193 = feedback #25() -> (w40:T11)
        n194 = Not Equal?(x=w41, y=w40) -> (x != y?=w42:bool)
        n195 = call-poly <vilib>:"PID.vi"("reinitialize? (F)"=w42, "output range"=w54, "PID gains"=w51, "process variable"=w52, "setpoint"=w53) -> ("output"=w36:dbl)  [unwired: 5 in, 1 out]
        n196 = call-poly <vilib>:"PID.vi"("reinitialize? (F)"=w42, "output range"=w44, "PID gains"=w45, "process variable"=w46, "setpoint"=w47) -> ("output"=w37:dbl)  [unwired: 5 in, 1 out]
        n197 = case shown="\"Kiwi Drive\"" w38 {
          tunnel: T16 {"Right"=0.0, "Left"=0.0, "Throttle"=0.0, "Wheel"=0.0, "Rotation"=0.0, "X"=0.0, "Y"=0.0} ("Drive Values") -> [w71 w75 _ _]
          tunnel: w37 -> [w68 w73 _ _]
          tunnel: w36 -> [w69 w74 _ _]
          tunnel: [w70 w72 T16 {"Right"=0.0, "Left"=0.0, "Throttle"=0.0, "Wheel"=0.0, "Rotation"=0.0, "X"=0.0, "Y"=0.0} ("Drive Values") T16 {"Right"=0.0, "Left"=0.0, "Throttle"=0.0, "Wheel"=0.0, "Rotation"=0.0, "X"=0.0, "Y"=0.0} ("Drive Values")] -> w35
          frame "Tank Drive 2 Motor", Default {
            n198 = Bundle By Name(cluster=w71, "Throttle"=w69, "Wheel"=w68) -> (w70:T16)
          }
          frame "Tank Drive 4 Motor" {
            n199 = Bundle By Name(cluster=w75, "Throttle"=w74, "Wheel"=w73) -> (w72:T16)
          }
          frame "Mecanum Drive" {
          }
          frame "Kiwi Drive" {
          }
        }
      }
    }
    n200 = node-c288(w17) -> ()  [unwired: 1 out]
  }
  n201 = node-c288(w7) -> ()  [unwired: 1 out]
